vi "Test_WriteValue_InvalidType_Error.vi"(8 "error in (no error)":errorcluster, 11 "TestCase in":refnum<class "TestBooleanTextBinding.lvclass">) -> (0 "error out":errorcluster, 3 "TestCase out":refnum<class "TestBooleanTextBinding.lvclass">)   [LabVIEW 2017, in "TestBooleanTextBinding.lvclass"]
uses:
  TestBooleanTextBinding.lvclass
  Source/Concrete/BooleanTextBinding/BooleanTextBinding.lvclass/BooleanTextBinding.ctl
  Source/Concrete/BooleanTextBinding/BooleanTextBinding.lvclass
  C:/Git/composed-transport/Source/ITransport/ITransport.lvclass
  <vilib>/Utility/error.llb/Error Cluster From Error Code.vi
  Source/ITransport/ITransport.lvclass
panel:
  in  "OK Button":bool
  out "Return Error":errorcluster
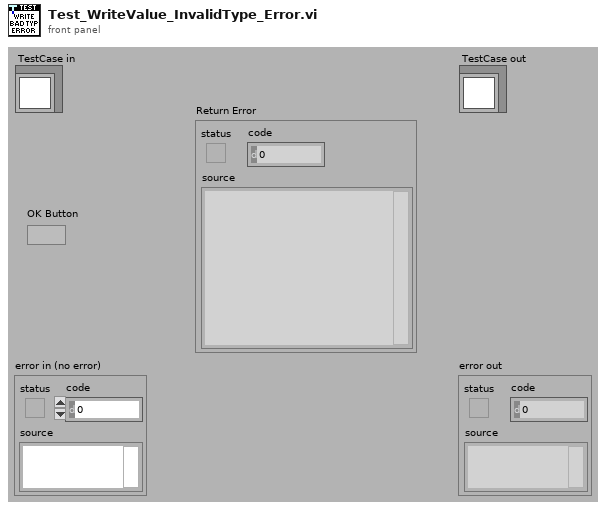
[diagram p1: front panel]
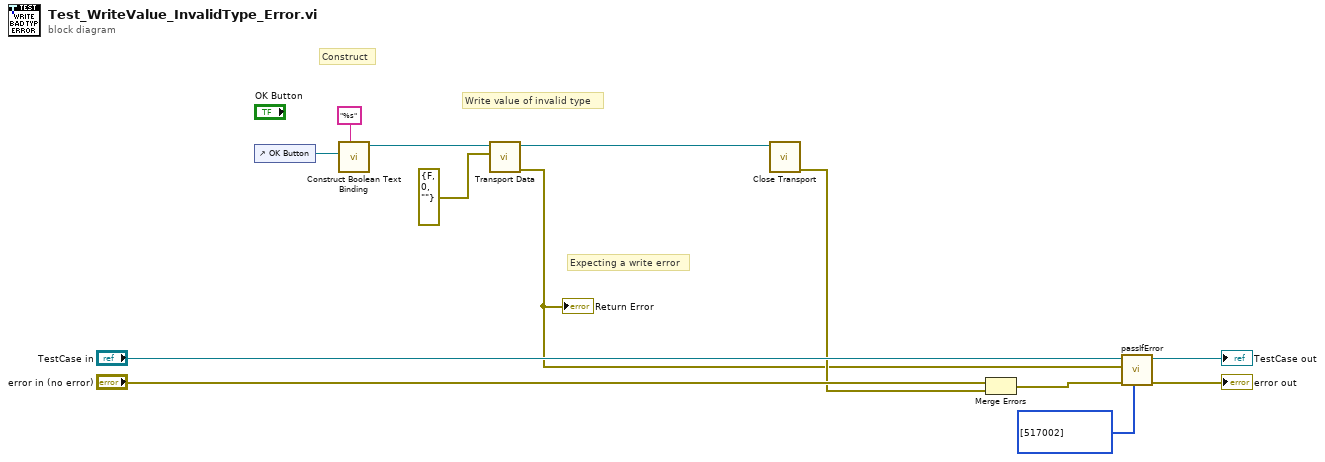
[diagram p0: block diagram]
diagram:
  # "Expecting a write error"
  # "Construct"
  # "Write value of invalid type"
  n1 = control-ref of="OK Button"() -> (w1:refnum<vi>)
  n2 = call "Construct Boolean Text Binding.vi"("Format String"="%s", "Bool Refnum"=w1) -> ("BooleanTextBinding"=w9:refnum<class "BooleanTextBinding.lvclass">)  [unwired: 8 in, 1 out]
  n3 = call "Transport Data.vi"("Value"=errorcluster {"status"=FALSE, "code"=0, "source"=""} ("error constant"), "ITransport in"=w9) -> ("error out"=w4:errorcluster, "ITransport out"=w7:refnum<class "BooleanTextBinding.lvclass">)  [unwired: 8 in]
  "Return Error" <- w4
  n4 = call-dynamic "Close Transport.vi"("ITransport in"=w7) -> ("error out"=w6:errorcluster)  [unwired: 10 in]
  n5 = Merge Errors("error in (no error)", w6) -> (w8:errorcluster)
  n6 = call-dynamic "passIfError.vi"("passing error codes (default = any error code)"=i32[] [517002], "error in (no error)"=w8, "error"=w4, "TestCase in"="TestCase in") -> ("error out"=→"error out":errorcluster, "TestCase out"=→"TestCase out":refnum<class "TestBooleanTextBinding.lvclass">)  [unwired: 6 in]
